vi "Deserialise content.vi"(8 "error in (no error)":errorcluster, 10 "JSON String to decode":string, 11 "object in":refnum<class "stream Message.lvclass">) -> (0 "error out":errorcluster, 3 "object out":refnum<class "stream Message.lvclass">)   [LabVIEW 2018, in "ClientMessaging.lvlib" / "stream Message.lvclass"]
doc: "Convert content dictionary to class private data"
uses:
  stream Message.lvclass
  19d44d0a-8435-463d-b959-4cf85a953d7b.vi
  3dd566e1-60c4-4f5d-9261-cd1ed0aa89ef.vi
  Base Classes/Message Class/Message Class.lvclass
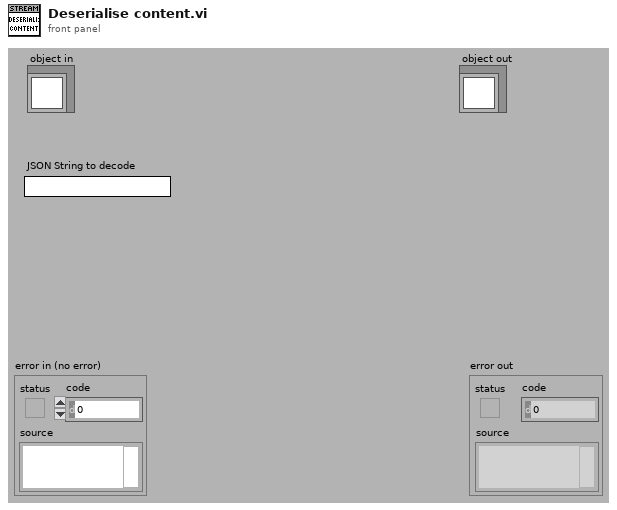
[diagram p1: front panel]
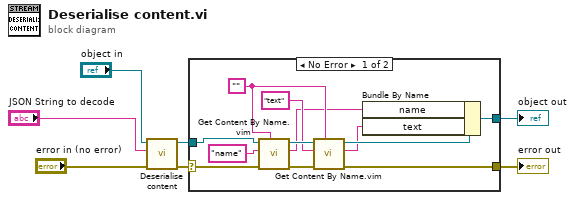
[diagram p0: block diagram]
diagram:
  n1 = call-parent "Deserialise content.vi"("error in (no error)"="error in (no error)", "JSON String to decode"="JSON String to decode", "object in"="object in") -> ("error out"=w1:errorcluster, "object out"=w4:refnum<class "stream Message.lvclass">)  [unwired: 7 in]
  n2 = case shown="No Error" w1 {
    selector: w1 -> [w8 w21]
    tunnel: [w15 w21] -> w7
    tunnel: [w19 w20] -> w5
    tunnel: w4 -> [w9 w20]
    frame No Error {
      w13 = ""
      n3 = call "Get Content By Name.vim"("Type of content"=w13, "error in (no error)"=w8, "Name of Content Item"="name", "Message In"=w9) -> ("error out"=w16:errorcluster, "Data Out"=w10:string, "Message Out"=w18:refnum<class "stream Message.lvclass">)  [unwired: 5 in]
      n4 = call "Get Content By Name.vim"("Type of content"=w13, "error in (no error)"=w16, "Name of Content Item"="text", "Message In"=w18) -> ("error out"=w15:errorcluster, "Data Out"=w11:string, "Message Out"=w17:refnum<class "stream Message.lvclass">)  [unwired: 5 in]
      n5 = Bundle By Name(cluster=w17, "name"=w10, "text"=w11) -> (w19:refnum<class "stream Message.lvclass">)
    }
    frame Error {
    }
  }
  "error out" <- w7
  "object out" <- w5
